vi "Solution part 1.vi"(11 "data?":bool) -> (3 "result":i32)   [LabVIEW 2020]
panel:
  out "diff as":i32
  out "orig as":i32
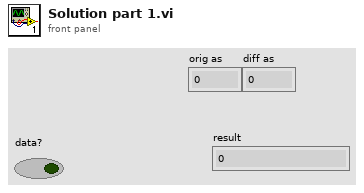
[diagram p1: front panel]
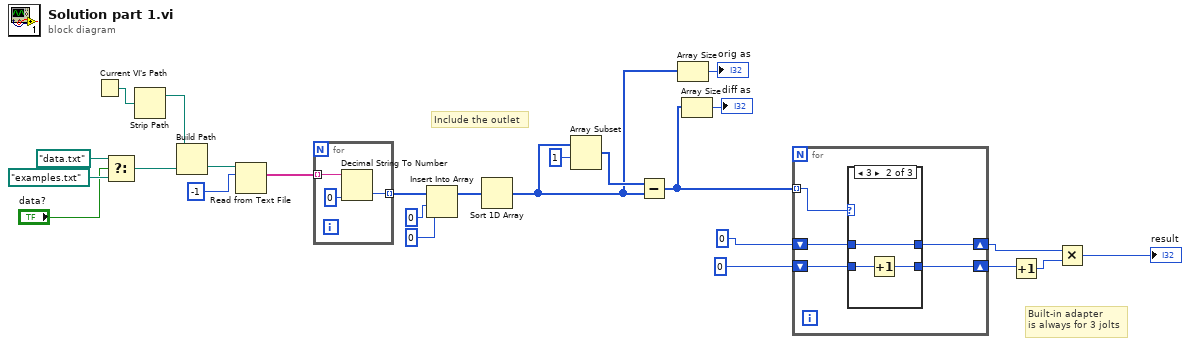
[diagram p0: block diagram]
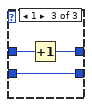
[diagram p3: hidden frame]
diagram:
  # "Include the outlet"
  # "Built-in adapter\nis always for 3 jolts"
  n1 = Current VI's Path() -> (path=w22:path)
  n2 = Select(t=path "data.txt", s="data?", f=path "examples.txt") -> (s? t:f=w23:path)
  n3 = Strip Path(path=w22) -> (stripped path=w21:path)  [unwired: 1 out]
  n4 = Build Path(base path=w21, name or relative path=w23) -> (appended path=w20:path)
  n5 = Read from Text File(file (use dialog)=w20, count=-1) -> (text=w17:string[])  [unwired: 2 in, 3 out]
  n6 = for {
    tunnel: w17 -> [w28] mode=indexing
    tunnel: [w26] -> w4 mode=indexing
    n7 = Decimal String To Number(string=w28, default (0L)=u64 0 ("count")) -> (number=w26:u64)  [unwired: 1 in, 1 out]
  }
  n8 = Insert Into Array(array=w4, index=0, new element=u64 0 ("new element/subarray")) -> (w3:u64[])
  n9 = Sort 1D Array(array=w3) -> (sorted array=w14:u64[])
  n10 = Array Subset(array=w14, index=1) -> (w15:u64[])  [unwired: 1 in]
  n11 = Subtract(x=w15, y=w14) -> (x-y=w11:u64[])
  n12 = Array Size(array=w14) -> (size(s)=→"orig as":i32)
  n13 = Array Size(array=w11) -> (size(s)=→"diff as":i32)
  n14 = for {
    tunnel: w11 -> [w29] mode=indexing
    shift-right: [w33] -> w6
    shift-left: 0 ("index") -> [w32]
    shift-right: [w31] -> w8
    shift-left: 0 ("index") -> [w30]
    n15 = case shown="3" w29 {
      tunnel: [w35 w38 w39] -> w33
      tunnel: w32 -> [w35 w38 w41]
      tunnel: [w34 w36 w40] -> w31
      tunnel: w30 -> [w34 w37 w40]
      frame Default {
      }
      frame 3 {
        n16 = Increment(x=w37) -> (x+1=w36:i32)
      }
      frame 1 {
        n17 = Increment(x=w41) -> (x+1=w39:i32)
      }
    }
  }
  n18 = Increment(x=w8) -> (x+1=w7:i32)
  n19 = Multiply(x=w6, y=w7) -> (x*y=→"result":i32)
